vi "Manuelno_Mjerenje.vi"() -> ()   [LabVIEW 2013]
panel:
  out "Waveform Chart 2":dynamicdata(graph)
  out "Waveform Chart":dynamicdata(graph)
  out "Numeric Indicator":dbl
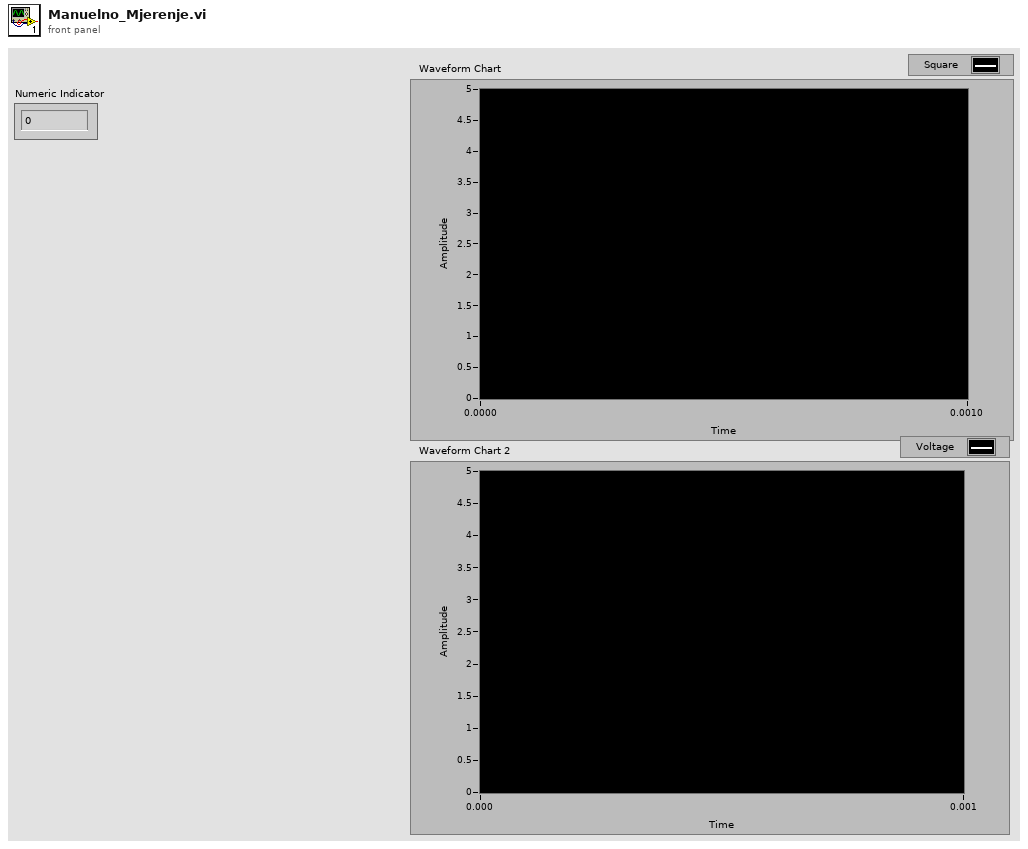
[diagram p1: front panel]
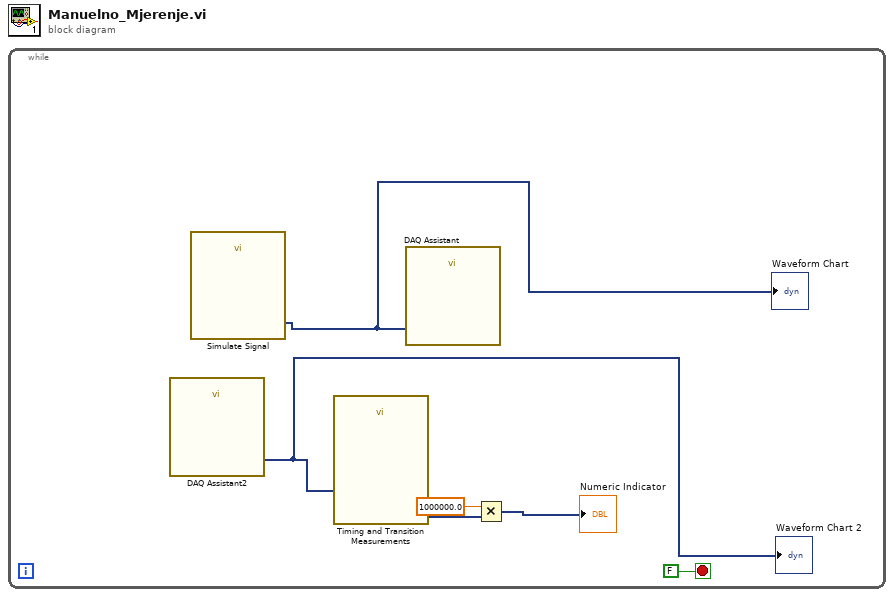
[diagram p0: block diagram]
diagram:
  n1 = while {
    stop <- FALSE stop-if-true
    n2 = call "DAQ Assistant2"() -> ("data"=w1:dynamicdata)  [unwired: 17 in, 2 out]
    "Waveform Chart 2" <- w1
    n3 = call "Simulate Signal"() -> ("Square"=w2:dynamicdata)  [unwired: 14 in, 1 out]
    "Waveform Chart" <- w2
    n4 = call "Timing and Transition Measurements"("Signals"=w1) -> ("Duration"=w5:dynamicdata)  [unwired: 9 in, 1 out]
    n5 = call "DAQ Assistant"("data"=w2) -> ()  [unwired: 16 in, 3 out]
    n6 = Multiply(x=1000000.0, y=w5) -> (x*y=→"Numeric Indicator":dynamicdata)
  }
